vi "UDT_application_UserEventsFGV.vi"() -> (3 "Unit Test Framework Results":T1)   [LabVIEW 2017]
doc: "Use this template to create a user-defined test VI. Define your test requirements and wire the results to the <b>Result (Test)</b> control. Do not modify the <b>Unit Test Framework Results</b> indicator."
uses:
  <vilib>/utf/common/utf_test_result_troll.ctl
  <vilib>/utf/common/utf_test_result.ctl
  <vilib>/utf/common/utf_test_result_failure.ctl
  <vilib>/utf/common/utf_test_comparison_operators.ctl
  <vilib>/utf/common/utf_vi_tag.ctl
  RT/UEFGV/Type Def/UEFGV_States.ctl
  <vilib>/event_ctls.llb/usereventprio.ctl
  <vilib>/Control Software Solutions Ltd/UTF Helper/SubVIs/UTF I32 Equals.vi
  <vilib>/Control Software Solutions Ltd/UTF Helper/Unit Test Helper.lvlib
  <vilib>/utf/NI_UnitTestFramework.lvlib
panel:
  out "Shutdown 2":bool
  out "Shutdown":bool
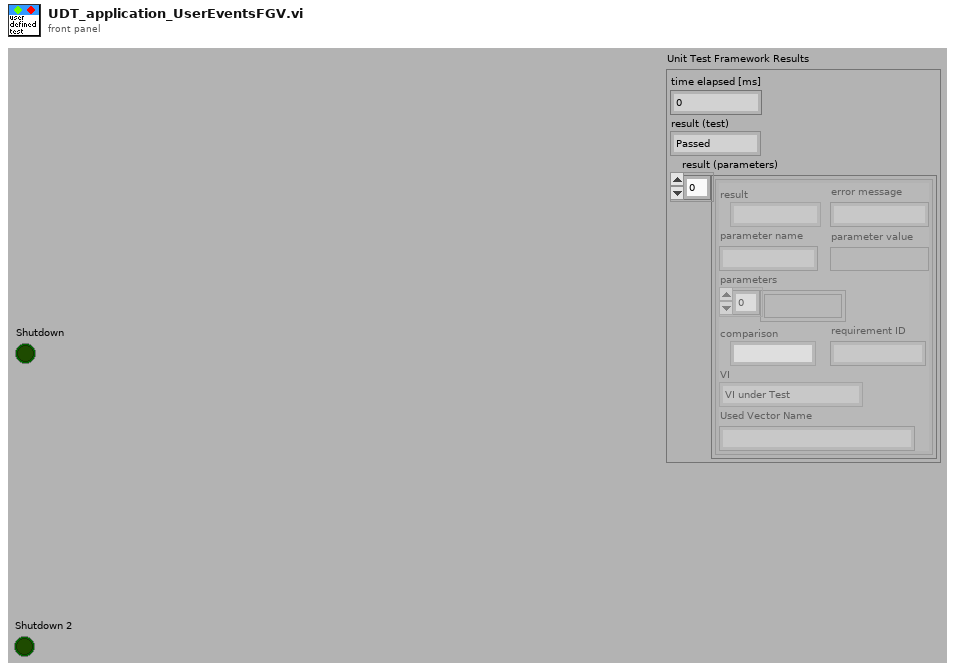
[diagram p1: front panel]
types:
  T1 = typedef "NI_UnitTestFramework.lvlib/utf_test_result_troll.ctl" = cluster{"time elapsed [ms]":u32, "result (test)":T2, "result (parameters)":T3[]}
  T2 = typedef "NI_UnitTestFramework.lvlib/utf_test_result.ctl" = enum16{"Passed", "Failed", "Error", "Skipped", "Not Processed"}
  T3 = typedef "NI_UnitTestFramework.lvlib/utf_test_result_failure.ctl" = cluster{"result":T2, "error message":string, "parameter name":string, "parameter value":variant, "parameters":variant[], "comparison":T4, "requirement ID":string, "VI":T5, "Used Vector Name":string}
  T4 = typedef "NI_UnitTestFramework.lvlib/utf_test_comparison_operators.ctl" = enum16{"=", "!=", ">", ">=", "<", "<=", "range", "symmetric tolerance", "asymmetric tolerance", "string contains", "string not contain", "array size", "string length", "array range", "by element", "array range (limit array)", "user-defined", "array contains", "array not contain", "vector length", "= (elm)", "!= (elm)", "= (case insensitive)", "!= (case insensitive)"}
  T5 = typedef "NI_UnitTestFramework.lvlib/utf_vi_tag.ctl" = enum16{"Setup VI", "VI under Test", "Teardown VI"}
  T6 = typedef "UEFGV_States.ctl" = enum16{"Create", "Get", "Destroy"}
  T7 = typedef "usereventprio.ctl" = enum32{"high priority", "normal priority"}
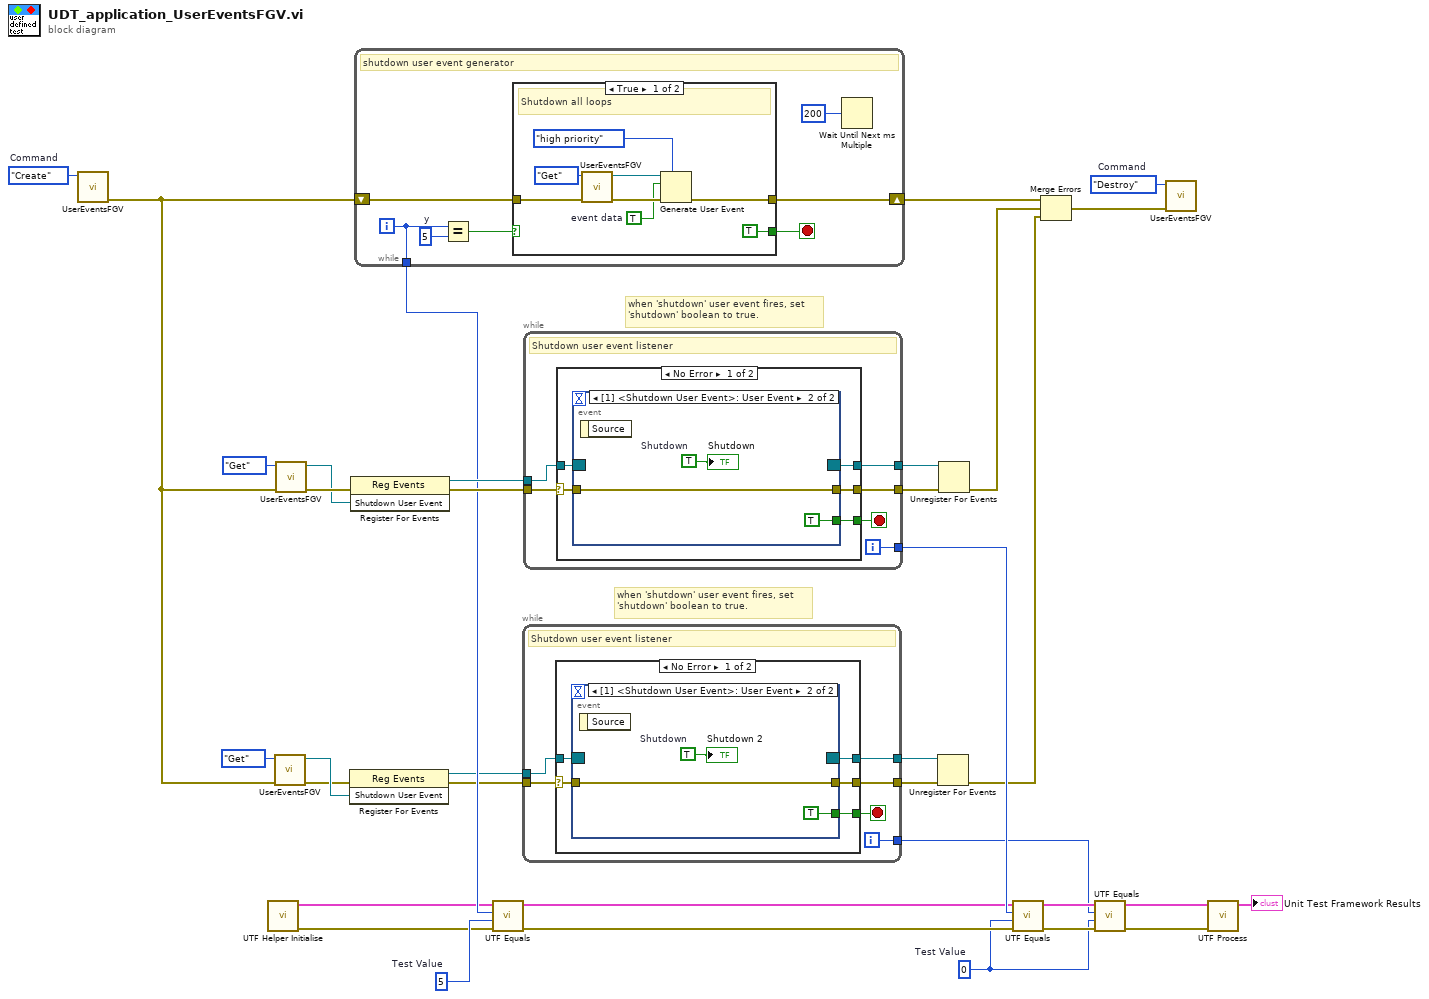
[diagram p0: block diagram]
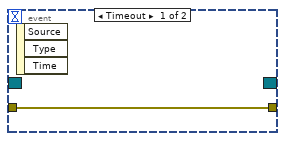
[diagram p2: hidden frame]
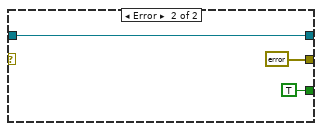
[diagram p3: hidden frame]
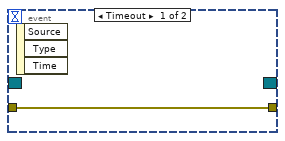
[diagram p4: hidden frame]
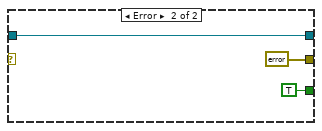
[diagram p5: hidden frame]
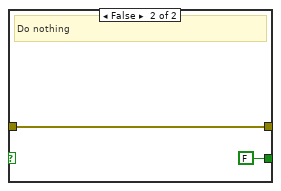
[diagram p6: hidden frame]
diagram:
  w18 = 5  # Test Value
  w4 = 0  # Test Value
  w24 = UEFGV_States."Destroy"  # Command
  w35 = UEFGV_States."Create"  # Command
  # "when 'shutdown' user event fires, set\n'shutdown' boolean to true."
  # "when 'shutdown' user event fires, set\n'shutdown' boolean to true."
  n1 = call "UserEventsFGV.vi"("Command"=w35) -> ("error out"=w8:errorcluster)  [unwired: 9 in, 1 out]
  n2 = call <vilib>:"UTF Helper Initialise.vi"() -> ("error out"=w16:errorcluster, "results array"=w17:T3[])  [unwired: 10 in]
  n3 = call "UserEventsFGV.vi"("error in (no error)"=w8, "Command"=UEFGV_States."Get") -> ("error out"=w11:errorcluster, "Shutdown User Event"=w12:refnum<user-event>)  [unwired: 8 in]
  n4 = call "UserEventsFGV.vi"("error in (no error)"=w8, "Command"=UEFGV_States."Get") -> ("error out"=w32:errorcluster, "Shutdown User Event"=w31:refnum<user-event>)  [unwired: 8 in]
  n5 = register-events(error in=w11, w12) -> (reference out=w9:refnum<event-registration>, error out=w14:errorcluster)  [unwired: 1 in]
  n6 = register-events(error in=w32, w31) -> (reference out=w34:refnum<event-registration>, error out=w29:errorcluster)  [unwired: 1 in]
  n7 = while {
    shift-right: [w39] -> w27
    shift-left: w8 -> [w40]
    tunnel: [w36] -> w19
    i -> [w36]
    stop <- w41 stop-if-true
    w38 = 5  # y
    # "shutdown user event generator"
    n8 = Equal?(x=w36, y=w38) -> (x = y?=w37:bool)
    n9 = case shown="True" w37 {
      tunnel: [TRUE FALSE] -> w41
      tunnel: w40 -> [w49 w51]
      tunnel: [w46 w51] -> w39
      frame True {
        w44 = TRUE  # event data
        # "Shutdown all loops"
        n10 = call "UserEventsFGV.vi"("error in (no error)"=w49, "Command"=UEFGV_States."Get") -> ("error out"=w48:errorcluster, "Shutdown User Event"=w47:refnum<user-event>)  [unwired: 8 in]
        n11 = Generate User Event(priority (normal)=usereventprio."high priority", user event=w47, event data cluster=w44, error in=w48) -> (error out=w46:errorcluster)  [unwired: 1 out]
      }
      frame False {
        # "Do nothing"
      }
    }
    n12 = Wait Until Next ms Multiple(millisecond multiple=u32 200) -> ()  [unwired: 1 out]
  }
  n13 = call-poly <vilib>:"UTF Equals.vi"("error in (no error)"=w16, "Test Value"=w18, "Input"=w19, "Input Results"=w17) -> ("error out"=w20:errorcluster, "Output Results"=w21:T3[])  [unwired: 6 in]
  n14 = while {
    tunnel: w9 -> [w58]
    tunnel: [w57] -> w10
    tunnel: w14 -> [w55]
    tunnel: [w54] -> w13
    tunnel: [w53] -> w3
    i -> [w53]
    stop <- w56 stop-if-true
    # "Shutdown user event listener"
    n15 = case shown="No Error" w55 {
      selector: w55 -> [w60 _]
      tunnel: w58 -> [w63 w69]
      tunnel: [w62 w69] -> w57
      tunnel: [w61 TRUE] -> w56
      tunnel: [w59 errorcluster {"status"=FALSE, "code"=0, "source"=""} ("error out")] -> w54
      frame No Error {
        n16 = event shown="[1] <Shutdown User Event>: User Event" {
          selector: w63 -> [_ _]
          dyn-events: [_ _] -> w62
          timeout: _ -> [_ _]
          tunnel: w60 -> [w64 w66]
          tunnel: [w64 w66] -> w59
          tunnel: [_ TRUE] -> w61
          event Timeout {
            n17 = event-data() -> ()  [unwired: 1 in, 3 out]
          }
          event User Event {
            w65 = TRUE  # Shutdown
            n18 = event-data() -> ()  [unwired: 1 in, 1 out]
            "Shutdown 2" <- w65
          }
        }
      }
      frame Error {
      }
    }
  }
  n19 = while {
    tunnel: w34 -> [w76]
    tunnel: [w75] -> w33
    tunnel: w29 -> [w73]
    tunnel: [w72] -> w30
    tunnel: [w71] -> w22
    i -> [w71]
    stop <- w74 stop-if-true
    # "Shutdown user event listener"
    n20 = case shown="No Error" w73 {
      selector: w73 -> [w78 _]
      tunnel: w76 -> [w81 w87]
      tunnel: [w80 w87] -> w75
      tunnel: [w79 TRUE] -> w74
      tunnel: [w77 errorcluster {"status"=FALSE, "code"=0, "source"=""} ("error out")] -> w72
      frame No Error {
        n21 = event shown="[1] <Shutdown User Event>: User Event" {
          selector: w81 -> [_ _]
          dyn-events: [_ _] -> w80
          timeout: _ -> [_ _]
          tunnel: w78 -> [w82 w84]
          tunnel: [w82 w84] -> w77
          tunnel: [_ TRUE] -> w79
          event Timeout {
            n22 = event-data() -> ()  [unwired: 1 in, 3 out]
          }
          event User Event {
            w83 = TRUE  # Shutdown
            n23 = event-data() -> ()  [unwired: 1 in, 1 out]
            "Shutdown" <- w83
          }
        }
      }
      frame Error {
      }
    }
  }
  n24 = Unregister For Events(event registration refnum=w10, error in=w13) -> (error out=w7:errorcluster)
  n25 = Unregister For Events(event registration refnum=w33, error in=w30) -> (error out=w26:errorcluster)
  n26 = call-poly <vilib>:"UTF Equals.vi"("error in (no error)"=w20, "Test Value"=w4, "Input"=w22, "Input Results"=w21) -> ("error out"=w5:errorcluster, "Output Results"=w6:T3[])  [unwired: 6 in]
  n27 = Merge Errors(w27, w26, w7) -> (w25:errorcluster)
  n28 = call-poly <vilib>:"UTF Equals.vi"("error in (no error)"=w5, "Test Value"=w4, "Input"=w3, "Input Results"=w6) -> ("error out"=w1:errorcluster, "Output Results"=w2:T3[])  [unwired: 6 in]
  n29 = call "UserEventsFGV.vi"("error in (no error)"=w25, "Command"=w24) -> ()  [unwired: 8 in, 2 out]
  n30 = call <vilib>:"UTF Process.vi"("error in (no error)"=w1, "results array"=w2) -> ("Unit Test Framework Results"=→"Unit Test Framework Results":T1)  [unwired: 9 in]
